vi "ATF Storage-AI C Start.vi"(8 "error in":errorcluster, 10 "AI C":T1(array[cluster]), 11 "Refnum in":refnum<k21>) -> (0 "error out":errorcluster, 3 "Refnum out":refnum<k21>)   [LabVIEW 2022 SP3]
uses:
  <vilib>/DAQmx/configure/timing.llb/DAQmx Timing (Sample Clock).vi
  <vilib>/DAQmx/configure/trigger.llb/DAQmx Start Trigger (Digital Edge).vi
  <resource>/objmgr/daqmx.rc
panel:
  in  "AI.DigFltr.Response 2":i32(ring)=10191 items=["Constant Group Delay"=16075, "Butterworth"=16076, "Elliptical"=16077, "Hardware Defined"=10191]
  in  "AI.DigFltr.Type 2":i32(ring)=16071 items=["Lowpass"=16071, "Highpass"=16072, "Bandpass"=16073, "Notch"=16074, "Custom"=10137]
  in  "AI.DigFltr.Lowpass.CutoffFreq 2":dbl=20.0
  in  "AI.DigFltr.Order 2":u32=4
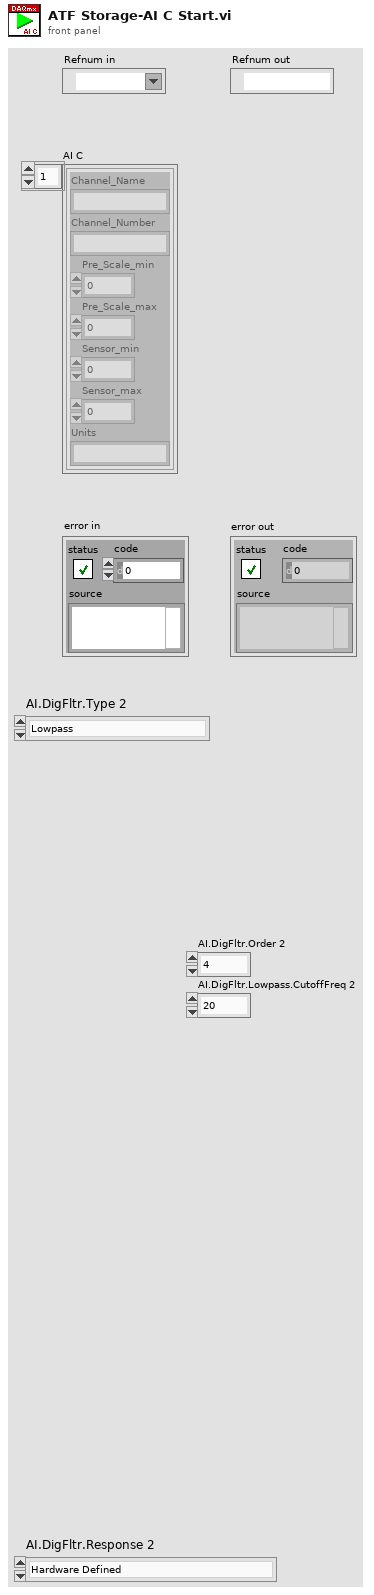
[diagram p1: front panel]
types:
  T1 = cluster{"Channel_Name":string, "Channel_Number":string, "Pre_Scale_min":dbl, "Pre_Scale_max":dbl, "Sensor_min":dbl, "Sensor_max":dbl, "Units":string}[]
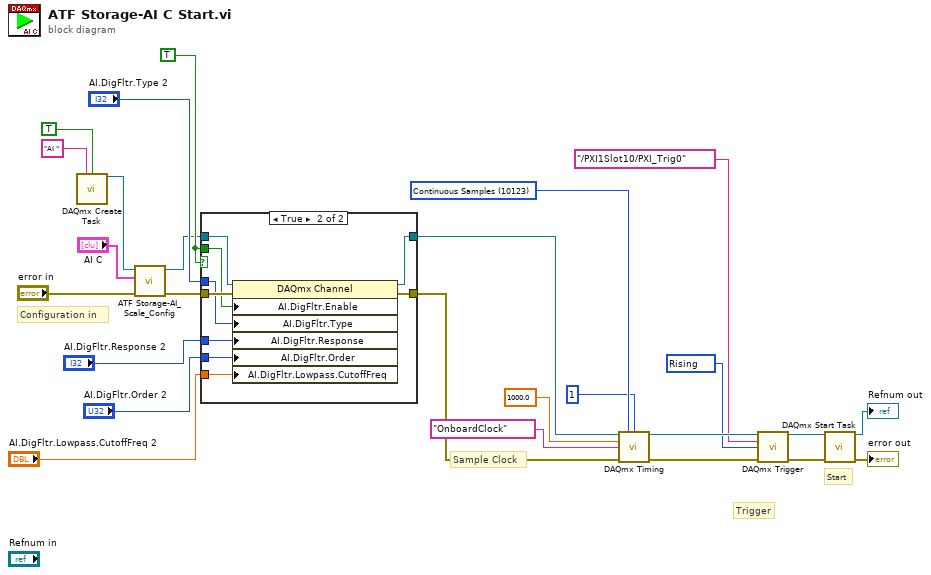
[diagram p0: block diagram]
diagram:
  w10 = TRUE
  w14 = 10280 items=["Rising"=10280, "Falling"=10171] ("edge")
  w22 = 10123 items=["Finite Samples"=10178, "Continuous Samples"=10123, "Hardware Timed Single Point"=12522] ("sample mode")
  # "Start"
  # "Trigger"
  # "Sample Clock"
  # "Configuration in"
  n1 = call <vilib>:"DAQmx Create Task.vi"("new task name"="AI ", "auto cleanup"=TRUE) -> ("task out"=w13:refnum<k21>)  [unwired: 12 in, 1 out]
  n2 = call "ATF Storage-AI_Scale_Config.vi"("error in (no error)"="error in", "AI C"="AI C", "Refnum in"=w13) -> ("error out"=w3:errorcluster, "Refnum out"=w5:refnum<k21>)  [unwired: 7 in]
  n3 = case shown="True" w10 {
    tunnel: w5 -> [w28 w37]
    tunnel: [w28 w36] -> w4
    tunnel: w3 -> [w27 w35]
    tunnel: [w27 w34] -> w2
    tunnel: w10 -> [_ w33]
    tunnel: "AI.DigFltr.Type 2" -> [_ w32]
    tunnel: "AI.DigFltr.Response 2" -> [_ w31]
    tunnel: "AI.DigFltr.Order 2" -> [_ w30]
    tunnel: "AI.DigFltr.Lowpass.CutoffFreq 2" -> [_ w29]
    frame False {
    }
    frame True {
      n4 = property class="DAQmx Channel"(reference=w37, error in=w35, "AI.DigFltr.Enable"=w33, "AI.DigFltr.Type"=w32, "AI.DigFltr.Response"=w31, "AI.DigFltr.Order"=w30, "AI.DigFltr.Lowpass.CutoffFreq"=w29) -> (reference out=w36:refnum<k21>, error out=w34:errorcluster)
    }
  }
  n5 = call-poly <vilib>:"DAQmx Timing.vi"("task/channels in"=w4, "sample mode"=w22, "samples per channel"=1, "rate"=1000.0, "source"=tag "OnboardClock", "error in"=w2) -> ("task out"=w25:refnum<k21>, "error out"=w16:errorcluster)  [unwired: 8 in]
  n6 = call-poly <vilib>:"DAQmx Trigger.vi"("task/channels in"=w25, "source"=tag "/PXI1Slot10/PXI_Trig0", "edge"=w14, "error in"=w16) -> ("task out"=w17:refnum<k21>, "error out"=w15:errorcluster)  [unwired: 10 in]
  n7 = call <vilib>:"DAQmx Start Task.vi"("task/channels in"=w17, "error in"=w15) -> ("task out"=→"Refnum out":refnum<k21>, "error out"=→"error out":errorcluster)  [unwired: 12 in]
